vi "project(3).vi"() -> ()   [LabVIEW 2009]
panel:
  in  "Password":string
  out "Armed in":i32
  in  "Front door initial":bool[](array[boolean])
  out "Front door indicator":bool[](array[boolean])
  in  "Window 1, window 2, back door 3 initially":bool[](array[boolean])
  in  "Window 1, window 2, back door 2":bool[](array[boolean])
  out "Alarm in":i32
  in  "Front door":bool[](array[boolean])
  out "Alarm":bool
  out "On indicates open":bool[](array[boolean])
  in  "Disarm":bool
  out "Armed":bool
  in  "?":bool
  # "Window 1"
  # "Window 2"
  # "Back door"
  # "Front door"
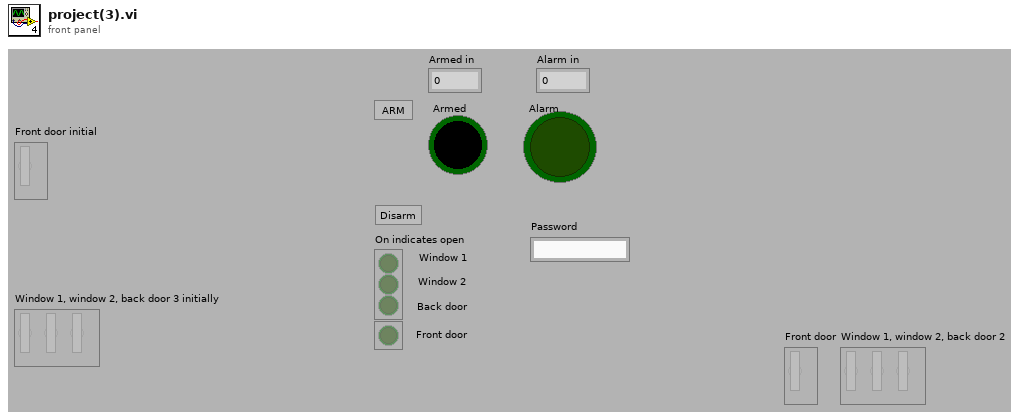
[diagram p1: front panel]
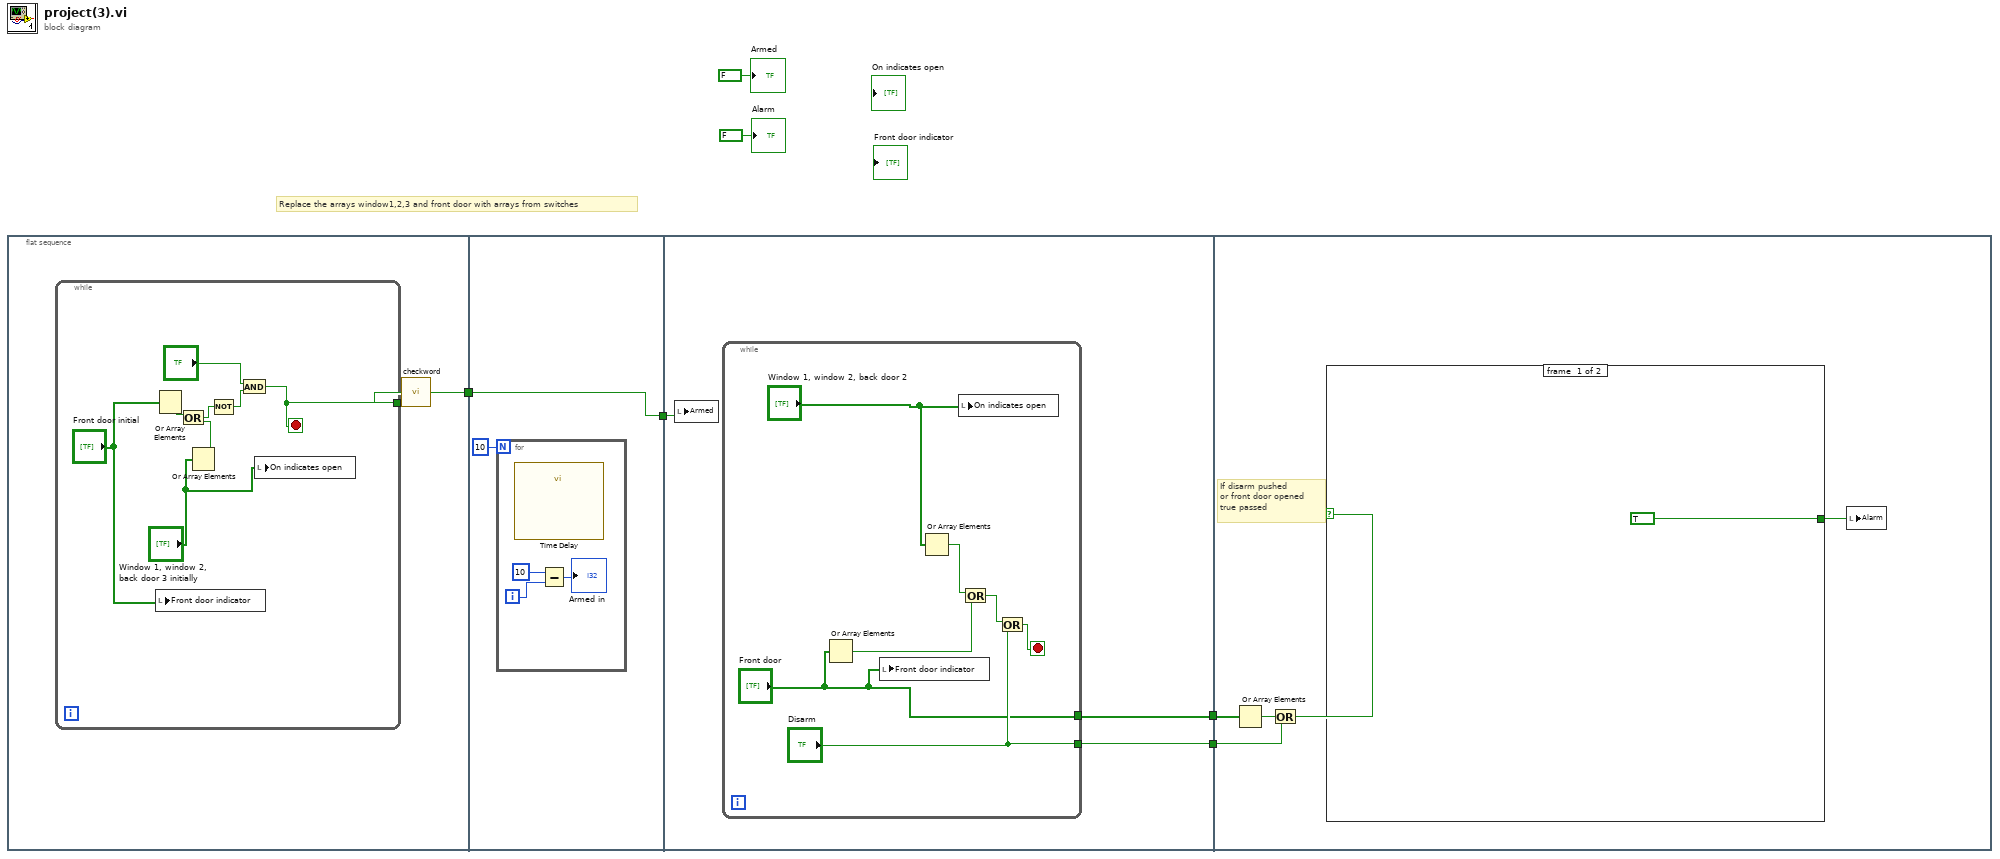
[diagram p0: block diagram]
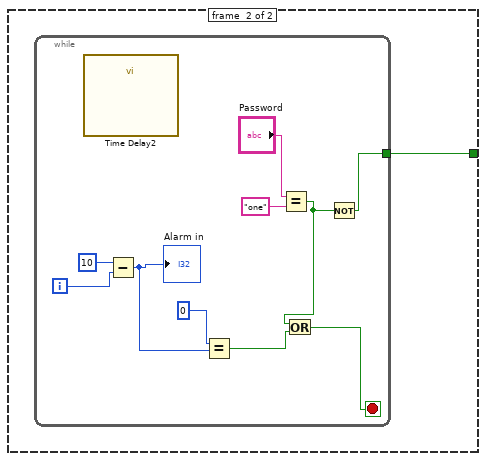
[diagram p2: hidden frame]
diagram:
  # "Replace the arrays window1,2,3 and front door with arrays from switches"
  n1 = flat-sequence {
    tunnel: [w7] -> w1
    tunnel: [w18] -> w2
    tunnel: w1 -> [w18]
    tunnel: [w24] -> w4
    tunnel: [w23] -> w3
    tunnel: w2 -> [w22]
    tunnel: w4 -> [w36]
    tunnel: w3 -> [w34]
    frame #0 {
      n2 = while {
        tunnel: [w15] -> w8
        stop <- w15 stop-if-true
        n3 = Or Array Elements(Boolean array="Front door initial") -> (logical OR=w11:bool)
        n4 = local write "Front door indicator"("Front door initial") -> ()
        n5 = Or Array Elements(Boolean array="Window 1, window 2, back door 3 initially") -> (logical OR=w10:bool)
        n6 = Or(x=w11, y=w10) -> (x .or. y?=w9:bool)
        n7 = Not(x=w9) -> (.not. x?=w14:bool)
        n8 = And(x="?", y=w14) -> (x .and. y?=w15:bool)
        n9 = local write "On indicates open"("Window 1, window 2, back door 3 initially") -> ()
      }
      n10 = call "checkword.vi"("Enable"=w8) -> ("Boolean"=w7:bool)
    }
    frame #1 {
      n11 = for {
        N: 10 -> [_]
        i -> [w21]
        n12 = call "Time Delay"() -> ()  [unwired: 11 in, 1 out]
        n13 = Subtract(x=10, y=w21) -> (x-y=→"Armed in":i32)
      }
    }
    frame #2 {
      n14 = local write "Armed"(w22) -> ()
      n15 = while {
        tunnel: ["Front door"] -> w24
        tunnel: ["Disarm"] -> w23
        stop <- w28 stop-if-true
        n16 = Or Array Elements(Boolean array="Front door") -> (logical OR=w30:bool)
        n17 = local write "Front door indicator"("Front door") -> ()
        n18 = Or Array Elements(Boolean array="Window 1, window 2, back door 2") -> (logical OR=w31:bool)
        n19 = local write "On indicates open"("Window 1, window 2, back door 2") -> ()
        n20 = Or(x=w31, y=w30) -> (x .or. y?=w29:bool)
        n21 = Or(x=w29, y="Disarm") -> (x .or. y?=w28:bool)
      }
    }
    frame #3 {
      # "If disarm pushed\nor front door opened\ntrue passed"
      n22 = Or Array Elements(Boolean array=w36) -> (logical OR=w35:bool)
      n23 = Or(x=w34, y=w35) -> (x .or. y?=w33:bool)
      n24 = case shown="True" w33 {
        tunnel: [TRUE ("Alarm") w38] -> w32
        frame #0 {
        }
        frame #1 {
          n25 = while {
            tunnel: [w39] -> w38
            i -> [w48]
            stop <- w41 stop-if-true
            n26 = call "Time Delay2"() -> ()  [unwired: 11 in, 1 out]
            n27 = Subtract(x=10, y=w48) -> (x-y=w46:i32)
            "Alarm in" <- w46
            n28 = Equal?(x=0, y=w46) -> (x = y?=w42:bool)
            n29 = Equal?(x="Password", y="one") -> (x = y?=w40:bool)
            n30 = Or(x=w40, y=w42) -> (x .or. y?=w41:bool)
            n31 = Not(x=w40) -> (.not. x?=w39:bool)
          }
        }
      }
      n32 = local write "Alarm"(w32) -> ()
    }
  }
  "Armed" <- FALSE ("Armed")
  "Alarm" <- FALSE ("Alarm")
